vi "Rst_Or.vi"(8 "error In":errorcluster, 9 "A*C rst":bool, 10 "L/Min rst":bool, 11 "BAR rst":bool) -> (0 "error out":errorcluster, 1 "A*C":bool, 2 "L/Min":bool, 3 "BAR":bool, 4 "Rst ind Color":cluster{u32, u32}[](array[cluster]), 5 "Rst":string)   [LabVIEW 2017]
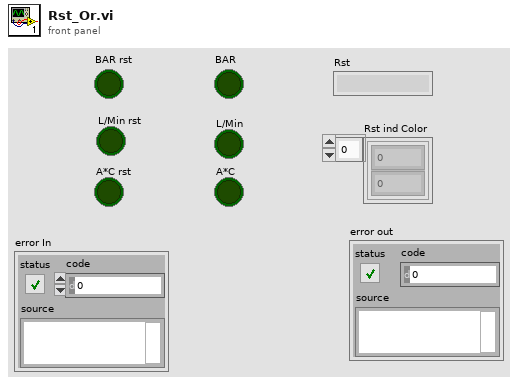
[diagram p1: front panel]
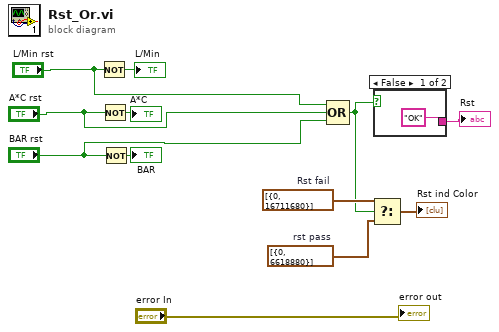
[diagram p0: block diagram]
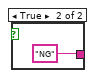
[diagram p2: hidden frame]
diagram:
  w11 = cluster{u32, u32}[] [{0, 6618880}]  # rst pass
  w12 = cluster{u32, u32}[] [{0, 16711680}]  # Rst fail
  n1 = Not(x="L/Min rst") -> (.not. x?=→"L/Min":bool)
  n2 = Not(x="A*C rst") -> (.not. x?=→"A*C":bool)
  n3 = Not(x="BAR rst") -> (.not. x?=→"BAR":bool)
  n4 = Compound Arithmetic op=OR("L/Min rst", "A*C rst", "BAR rst") -> (w7:bool)
  n5 = Select(t=w12, s=w7, f=w11) -> (s? t:f=→"Rst ind Color":cluster{u32, u32}[])
  n6 = case shown="False" w7 {
    tunnel: ["OK" "NG"] -> w6
    frame False {
    }
    frame True {
    }
  }
  "Rst" <- w6
  "error out" <- "error In"
